vi "Get to upper angle.vi"(2 "error in (no error)":errorcluster) -> (0 "error out":errorcluster)   [LabVIEW 2013]
uses:
  InTake Global Data.vi
  Cannon/Cannon Global Data.vi
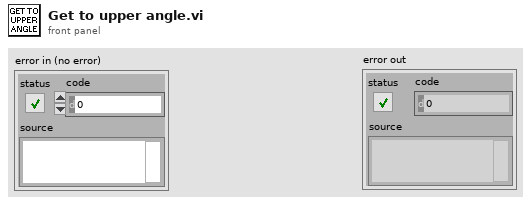
[diagram p1: front panel]
types:
  T1 = cluster{"TakeBall":dbl, "UpperClaw":dbl, "LowerClaw":dbl, "MS":bool, "Upper claw max":bool, "Lower claw max":bool, "Upper claw min":bool, "Lower claw min":bool, "Angle":dbl}
  T2 = typedef "WPI_SolenoidValue.ctl" = enum16{"Off", "On", "Forward", "Reverse"}
  T3 = cluster{"MS":bool, "Shoot!":T2, "Angle":dbl, "Reset Gyro?":bool}
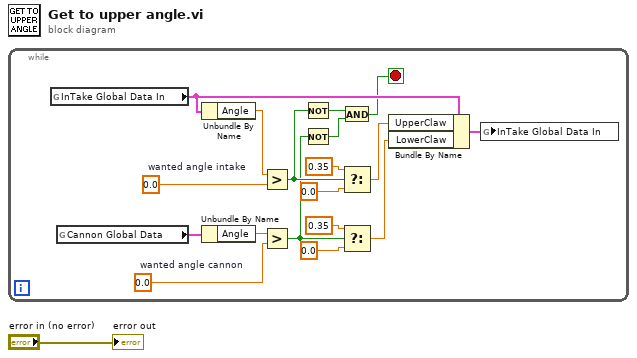
[diagram p0: block diagram]
diagram:
  n1 = while {
    stop <- w2 stop-if-true
    w10 = 0.0  # wanted angle cannon
    w15 = 0.0  # wanted angle intake
    n2 = global read "InTake Global Data.vi" "InTake Global Data In"() -> (w18:T1)
    n3 = global read "Cannon Global Data.vi" "Cannon Global Data"() -> (w17:T3)
    n4 = Unbundle By Name(w18) -> ("Angle"=w16:dbl)
    n5 = Unbundle By Name(w17) -> ("Angle"=w9:dbl)
    n6 = Greater?(x=w16, y=w15) -> (0:w6:bool)
    n7 = Greater?(x=w9, y=w10) -> (0:w5:bool)
    n8 = Not(x=w6) -> (.not. x?=w4:bool)
    n9 = Not(x=w5) -> (.not. x?=w3:bool)
    n10 = And(x=w4, y=w3) -> (x .and. y?=w2:bool)
    n11 = Select(t=0.35, s=w6, f=0.0) -> (s? t:f=w8:dbl)
    n12 = Select(t=0.35, s=w5, f=0.0) -> (s? t:f=w7:dbl)
    n13 = Bundle By Name(cluster=w18, "UpperClaw"=w8, "LowerClaw"=w7) -> (w19:T1)
    n14 = global write "InTake Global Data.vi" "InTake Global Data In"(w19) -> ()
  }
  "error out" <- "error in (no error)"
